vi "Configure Channel.vi"(8 "error in":errorcluster, 9 "Channel":u8=1 min=1 max=127 step=1, 11 "VISA resource name":refnum<visa-resource-name>) -> (0 "error out":errorcluster, 3 "VISA resource name out":refnum<visa-resource-name>)   [LabVIEW 2020, in "IT-M7700.lvlib"]
doc: "This command is used to set the address for the upper computer to transmit data to the on-line instrument.\n<b>Channel</b>\n1-127"
uses:
  <instrlib>/IT-M7700/IT-M7700.lvlib
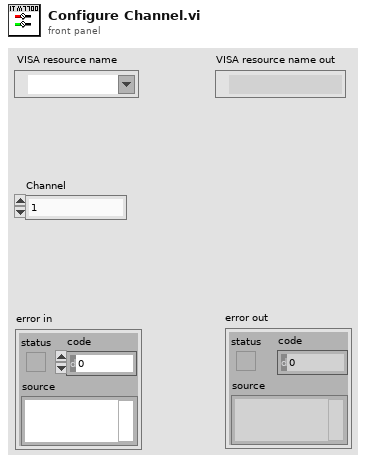
[diagram p1: front panel]
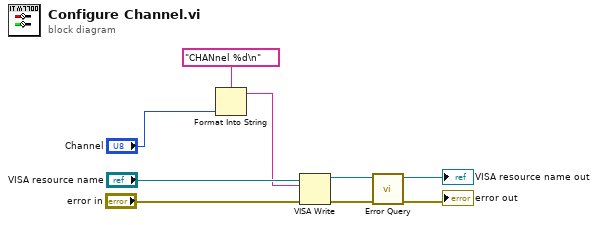
[diagram p0: block diagram]
diagram:
  n1 = Format Into String(format string="CHANnel %d\n", "Channel") -> (resulting string=w6:string)  [unwired: 2 in, 1 out]
  n2 = VISA Write(VISA resource name="VISA resource name", write buffer=w6, error in (no error)="error in") -> (VISA resource name out=w5:refnum<visa-resource-name>, error out=w4:errorcluster)  [unwired: 1 out]
  n3 = call <instrlib>:"Error Query.vi"("error in"=w4, "VISA resource name"=w5) -> ("error out"=→"error out":errorcluster, "VISA resource name out"=→"VISA resource name out":refnum<visa-resource-name>)  [unwired: 6 in, 2 out]
